vi "Create Listener.vi"(8 "error in":errorcluster, 11 "TCP slave in":refnum<class "TCP Slave.lvclass">) -> (0 "error out":errorcluster, 3 "TCP slave out":refnum<class "TCP Slave.lvclass">)   [LabVIEW 2012, in "TCP Slave.lvclass"]
doc: "Creates a new listener on the stored port, and then stores that in the class."
uses:
  TCP Slave.lvclass
  TCP Slave.lvclass/TCP Slave.ctl
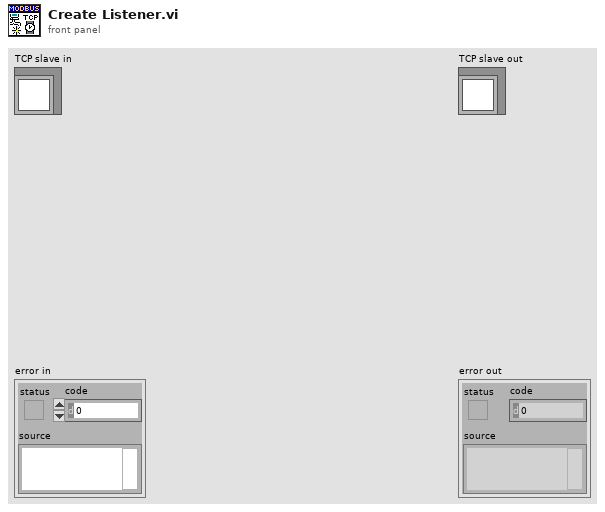
[diagram p1: front panel]
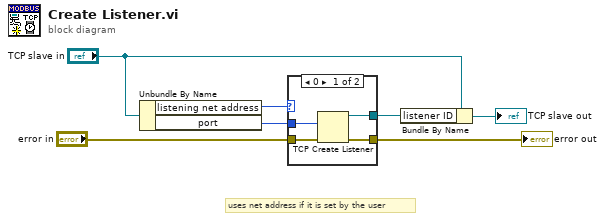
[diagram p0: block diagram]
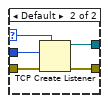
[diagram p2: hidden frame]
diagram:
  # "uses net address if it is set by the user"
  n1 = Unbundle By Name("TCP slave in") -> ("listening net address"=w1:u32, "port"=w3:u16)
  n2 = case shown="0" w1 {
    selector: w1 -> [_ w12]
    tunnel: "error in" -> [w11 w16]
    tunnel: [w9 w15] -> w6
    tunnel: w3 -> [w10 w14]
    tunnel: [w8 w13] -> w2
    frame 0 {
      n3 = TCP Create Listener(8:w11, 10:w10) -> (0:w9:errorcluster, 3:w8:refnum<k5>)  [unwired: 3 in, 1 out]
    }
    frame Default {
      n4 = TCP Create Listener(7:w12, 8:w16, 10:w14) -> (0:w15:errorcluster, 3:w13:refnum<k5>)  [unwired: 2 in, 1 out]
    }
  }
  "error out" <- w6
  n5 = Bundle By Name(cluster="TCP slave in", "listener ID"=w2) -> (→"TCP slave out":refnum<class "TCP Slave.lvclass">)
